vi "eraseAO_img.vi"   [LabVIEW 2015]
types:
  T1 = typedef "LVRectTypeDef.ctl" = cluster{"Left":i16, "Top":i16, "Right":i16, "Bottom":i16}
  T2 = cluster{"Xpixels":i32, "Vxminref":dbl, "Vxmaxref":dbl, "P":dbl, "Ypixels":i32, "Vyminref":dbl, "Vymaxref":dbl, "srate":sgl, "sAOxy":i32, "timeout":dbl, "type":string, "date":string, "time":string, "Colormap":u16, "Drawing Mode":u16, "Scanning Mode":u16, "square pixels":bool, "square matrix":bool, "Xpixels Img":i32, "Vx-min Img":dbl, "VX-max Img":dbl, "Ypixels Img":i32, "Vy-min Img":dbl, "Vy-max Img ":dbl, "Angle Img":dbl, "autoshutter":bool, "finite":bool, "cont":bool, "wavdet":bool, "measpoints":i32, "avpp":i32, "bufferAO":i32, "bufferAI":i32, "starttick":u32, "waveform":path, "Vx-ref":dbl, "Vy-ref":dbl, "refreshrate":dbl, "refreshbuffer":i32, "tt_cycles":i32, "motorref":refnum<k7>, "mirrorswitch":refnum<k7>, "sample mode":i32, "maxbufferAI":i32, "srateAODO":sgl, "bin":sgl, "Pel":sgl, "Angle draw":dbl, "srate Img":sgl, "ROIimg_plotbounds":T1, "auto OD":bool, "ODfilt":u16, "aAI":i32[], "aCI":i32[], "aAO":u32[], "aDO":u32[], "refwfsize":dbl, "Lifetime":bool, "Vz-Img":dbl, "Vz-ref":dbl, "Vz-reset":dbl, "AIoverride":bool}
  T3 = cluster{"AO":refnum<k21>[], "E_AO":errorcluster[]}
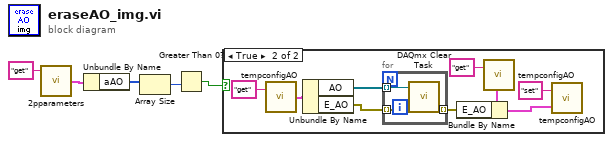
[diagram p0: block diagram]
diagram:
  n1 = call "2pparameters.vi"("command"="get") -> ("params out"=w4:T2)  [unwired: 1 in]
  n2 = Unbundle By Name(w4) -> ("aAO"=w3:u32[])
  n3 = Array Size(array=w3) -> (size(s)=w2:i32)
  n4 = Greater Than 0?(x=w2) -> (x > 0?=w1:bool)
  n5 = case shown="True" w1 {
    frame False {
    }
    frame True {
      n6 = call "tempconfigAO.vi"("command"="get") -> ("Temp Config out"=w13:T3)  [unwired: 1 in]
      n7 = Unbundle By Name(w13) -> ("AO"=w7:refnum<k21>[], "E_AO"=w6:errorcluster[])
      n8 = for {
        tunnel: [w17] -> w9 mode=indexing
        tunnel: w7 -> [w16] mode=indexing
        tunnel: w6 -> [w15] mode=indexing
        n9 = call <vilib>:"DAQmx Clear Task.vi"("task in"=w16, "error in"=w15) -> ("error out"=w17:errorcluster)  [unwired: 13 in]
      }
      n10 = call "tempconfigAO.vi"("command"="get") -> ("Temp Config out"=w10:T3)  [unwired: 1 in]
      n11 = Bundle By Name(cluster=w10, "E_AO"=w9) -> (w8:T3)
      n12 = call "tempconfigAO.vi"("Temp Config in"=w8, "command"="set") -> ()  [unwired: 1 out]
    }
  }
